vi "APLUS Camille Bauer Driver Tester.vi"() -> ()   [LabVIEW 2016]
panel:
  in  "stop":bool
  out "APLUS Data":string[][](array[string])
  in  "Remote Port":u16=502
  in  "Remote IP Address":string="10.0.3.101"
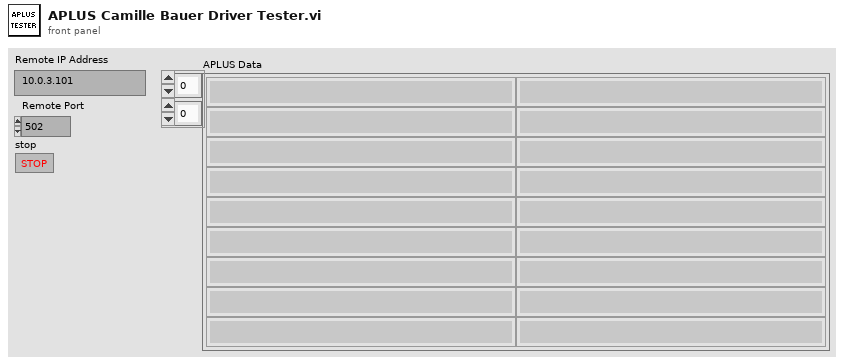
[diagram p1: front panel]
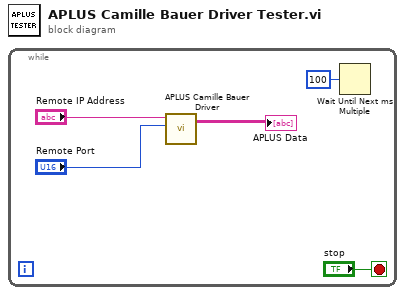
[diagram p0: block diagram]
diagram:
  n1 = while {
    stop <- "stop" stop-if-true
    n2 = call "APLUS Camille Bauer Driver.vi"("Remote Port"="Remote Port", "Remote IP Address"="Remote IP Address") -> ("APLUS Data"=→"APLUS Data":string[][])  [unwired: 5 in, 4 out]
    n3 = Wait Until Next ms Multiple(millisecond multiple=u32 100) -> ()  [unwired: 1 out]
  }
